vi "Test Disable Plugins.vi"(8 "error in (no error)":errorcluster, 11 "Configuration Manager Test in":refnum<class "Configuration Manager Test.lvclass">) -> (0 "error out":errorcluster, 3 "Configuration Manager Test out":refnum<class "Configuration Manager Test.lvclass">)   [LabVIEW 2020, in "Configuration Manager Test.lvclass"]
uses:
  Configuration Manager Test.lvclass
  C:/Program Files (x86)/National Instruments/LabVIEW 2020/vi.lib/Astemes/LUnit/Test Case.lvclass
  <vilib>/Astemes/LUnit/Test Case.lvclass/Test Case.ctl
  b78b68b9-28ec-4fcb-9b61-f705c7f0904e.vi
  <vilib>/Astemes/LUnit/Palette/Pass.vi
  <vilib>/Astemes/LUnit/Palette/Fail.vi
  <vilib>/Astemes/LUnit/Compare Variants.vi
  <vilib>/Astemes/LUnit/Describe Comparison.vi
  <vilib>/Astemes/LUnit/Set Assertion Type.vi
  <vilib>/Astemes/LUnit/Add test result.vi
  <vilib>/Astemes/LUnit/Variant to string.vi
  <vilib>/Astemes/LUnit/LUnit Record Assertion Result.vi
  <vilib>/Astemes/LUnit/LUnit Aggregate Assertion Results.vi
  <vilib>/Astemes/LUnit/Method Result/LUnit Merge Status.vi
  <vilib>/Astemes/LUnit/LUnit Concatenate result strings.vi
  <vilib>/Utility/Data Type/Get Type Information.vi
  <vilib>/Utility/LVClass/Get LV Class Name.vi
  source/User Interface/Configuration Manager/Configuration Manager.lvclass
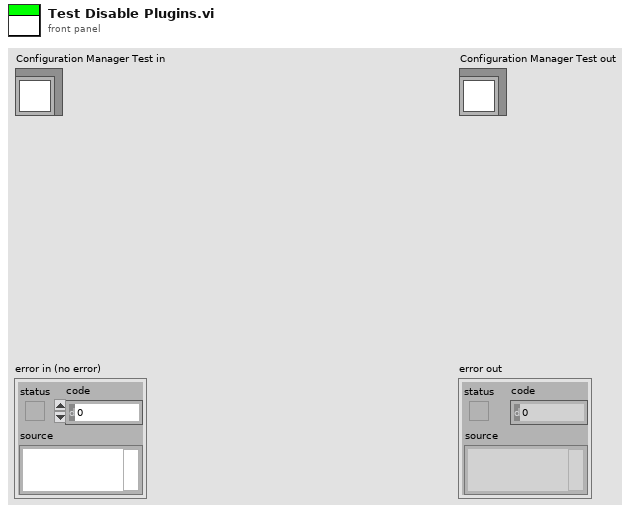
[diagram p1: front panel]
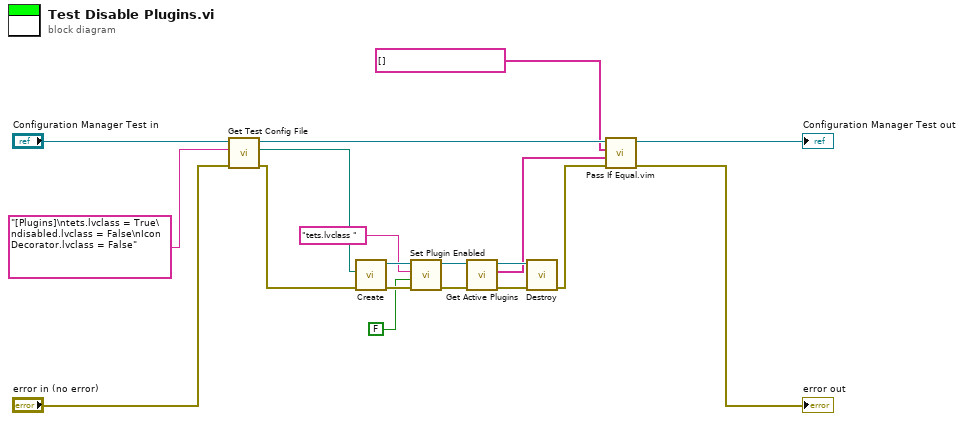
[diagram p0: block diagram]
diagram:
  n1 = call "Get Test Config File.vi"("error in (no error)"="error in (no error)", "File Content"="[Plugins]\ntets.lvclass = True\ndisabled.lvclass = False\nIcon Decorator.lvclass = False", "Configuration Manager Test in"="Configuration Manager Test in") -> ("error out"=w13:errorcluster, "File Path"=w8:path, "Configuration Manager Test out"=w10:refnum<class "Configuration Manager Test.lvclass">)  [unwired: 6 in]
  n2 = call "Create.vi"("error in (no error)"=w13, "configuration file path"=w8) -> ("error out"=w16:errorcluster, "Configuration Manager out"=w4:refnum<class "Configuration Manager.lvclass">)  [unwired: 8 in]
  n3 = call "Set Plugin Enabled.vi"("error in (no error)"=w16, "Enabled?"=FALSE, "Plugin"="tets.lvclass ", "Configuration Manager in"=w4) -> ("error out"=w5:errorcluster, "Configuration Manager out"=w3:refnum<class "Configuration Manager.lvclass">)  [unwired: 6 in]
  n4 = call "Get Active Plugins.vi"("error in (no error)"=w5, "Configuration Manager In"=w3) -> ("error out"=w14:errorcluster, "Plugins"=w7:string[], "Configuration Manager Out"=w15:refnum<class "Configuration Manager.lvclass">)  [unwired: 7 in]
  n5 = call "Destroy.vi"("error in (no error)"=w14, "Configuration Manager In"=w15) -> ("error out"=w12:errorcluster)  [unwired: 9 in]
  n6 = call "Pass If Equal.vim"("error in (no error)"=w12, "Actual"=w7, "Expected"=string[] [], "LUnit Test Case In"=w10) -> ("error out"=→"error out":errorcluster, "LUnit Test Case Out"=→"Configuration Manager Test out":refnum<class "Configuration Manager Test.lvclass">)  [unwired: 6 in]
